vi "写D+16位.vi"(8 "error out":errorcluster, 9 "输入数值":i32, 10 "输入地址D":i32, 11 "VISA resource name out":refnum<visa-resource-name>) -> (0 "error out 2":errorcluster caption="error out", 2 "通讯延时":u32, 3 "VISA resource name out 2":refnum<visa-resource-name>, 4 "连接的字符串":string, 5 "读取缓冲区":string)   [LabVIEW 2018]
uses:
  <vilib>/Instr/_visa.llb/VISA Configure Serial Port (Instr).vi
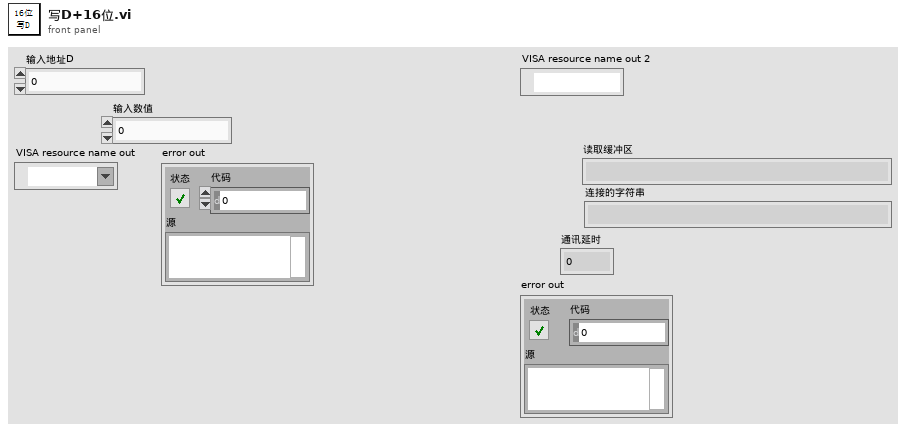
[diagram p1: front panel]
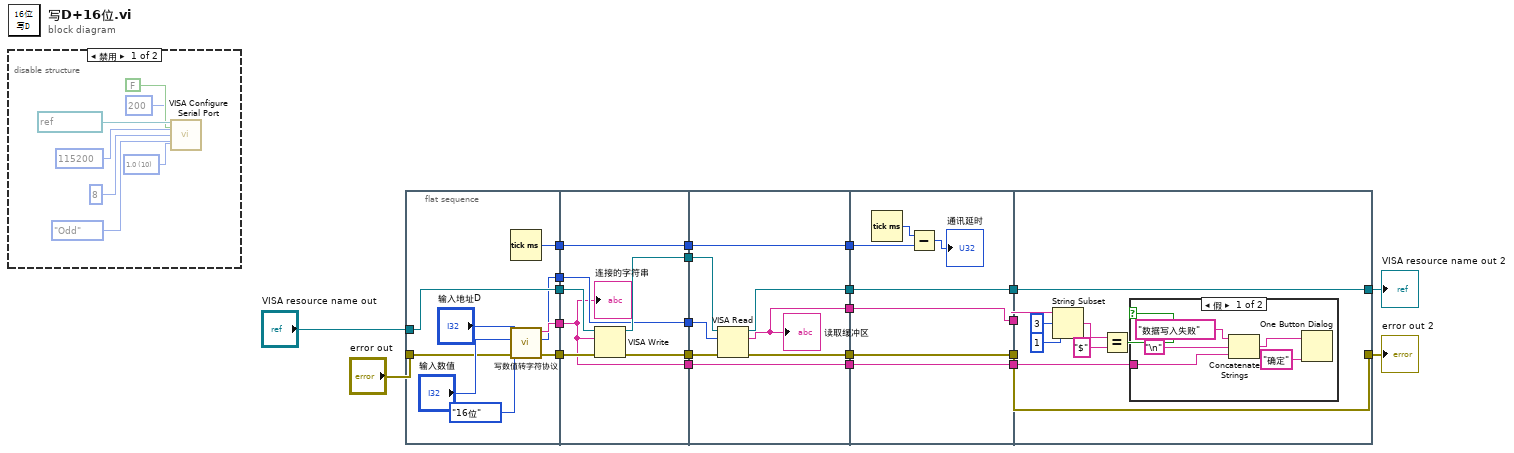
[diagram p0: block diagram]
diagram:
  n1 = disable-structure shown="禁用" {
    frame Disabled {
      w26 = u16 10 items=["1.0"=10, "1.5"=15, "2.0"=20] ("stop bits (10: 1 bit)")
      n2 = call-poly "VISA Configure Serial Port"("VISA resource name"=refnum<visa-resource-name> "COM3", "timeout (10sec)"=u32 200, "Enable Termination\nChar (T)"=FALSE ("Enable Termination\nChar (T)"), "baud rate (9600)"=u32 115200, "data bits (8)"=u16 8, "parity (0:none)"=enum16{"None", "Odd", "Even", "Mark", "Space"}."Odd", "stop bits (10: 1 bit)"=w26) -> ()  [unwired: 7 in, 2 out]
    }
    frame Enabled {
    }
  }
  n3 = flat-sequence {
    tunnel: "VISA resource name out" -> [w37]
    tunnel: "error out" -> [w36]
    tunnel: [w37] -> w23
    tunnel: [w36] -> w22
    tunnel: [w35] -> w21
    tunnel: [w34] -> w17
    tunnel: [w33] -> w16
    tunnel: w23 -> [w44]
    tunnel: w22 -> [w45]
    tunnel: w21 -> [w39]
    tunnel: [w43] -> w20
    tunnel: [w42] -> w19
    tunnel: [w41] -> w18
    tunnel: w17 -> [w41]
    tunnel: w16 -> [w40]
    tunnel: [w40] -> w15
    tunnel: [w39] -> w1
    tunnel: w20 -> [w51]
    tunnel: w19 -> [w50]
    tunnel: w18 -> [w49]
    tunnel: w15 -> [w48]
    tunnel: [w53] -> w14
    tunnel: [w52] -> w13
    tunnel: [w48] -> w12
    tunnel: [w47] -> w8
    tunnel: [w46] -> w2
    tunnel: w1 -> [w46]
    tunnel: w14 -> [w60]
    tunnel: w13 -> [w59]
    tunnel: w12 -> [w57]
    tunnel: [w60] -> w11
    tunnel: [w59] -> w10
    tunnel: [w55] -> w9
    tunnel: w8 -> [w55]
    tunnel: [w54] -> w3
    tunnel: w2 -> [w54]
    tunnel: [w68] -> w4
    tunnel: [w69] -> w5
    tunnel: w11 -> [w69]
    tunnel: w10 -> [w68]
    tunnel: w9 -> [w67]
    tunnel: w3 -> [w61]
    frame #0 {
      n4 = Tick Count (ms)() -> (millisecond timer value=w33:u32)
      n5 = call "写数值转字符协议.vi"("枚举"=enum16{"16位", "32位"}."16位", "输入数值"="输入数值", "输入地址"="输入地址D") -> ("返回字节数"=w34:u16, "连接的字符串"=w35:string)  [unwired: 7 in]
    }
    frame #1 {
      n6 = VISA Write(VISA resource name=w44, write buffer=w39, error in (no error)=w45) -> (VISA resource name out=w43:refnum<visa-resource-name>, error out=w42:errorcluster)  [unwired: 1 out]
      "连接的字符串" <- w39
    }
    frame #2 {
      n7 = VISA Read(VISA resource name=w51, byte count=w49, error in (no error)=w50) -> (VISA resource name out=w53:refnum<visa-resource-name>, read buffer=w47:string, error out=w52:errorcluster)  [unwired: 1 out]
      "读取缓冲区" <- w47
    }
    frame #3 {
      n8 = Tick Count (ms)() -> (millisecond timer value=w58:u32)
      n9 = Subtract(x=w58, y=w57) -> (x-y=→"通讯延时":u32)
    }
    frame #4 {
      n10 = String Subset(string=w67, offset (0)=3 ("偏移量(0)"), length (rest)=1 ("长度（剩余）")) -> (substring=w64:string)
      n11 = Equal?(x=w64, y="$") -> (x = y?=w62:bool)
      n12 = case shown="假" w62 {
        tunnel: w61 -> [w71 _]
        frame False {
          n13 = Concatenate Strings("数据写入失败" ("消息"), "\n", w71) -> (w70:string)
          n14 = One Button Dialog(message=w70, button name ("OK")="确定" ("按钮名称（“确定”）")) -> ()  [unwired: 1 out]
        }
        frame True {
        }
      }
    }
  }
  "VISA resource name out 2" <- w5
  "error out 2" <- w4
